vi "TestMotors.vi"() -> ()   [LabVIEW 2016]
uses:
  MotorControl/Configurations.ctl
  <vilib>/robotics/Steering/Wheel/Wheel Parameters.ctl
  <vilib>/robotics/Steering/Wheel/Rotation Direction.ctl
  <vilib>/Platform/TimedLoop/XDataNode/timing_clust.ctl
  <vilib>/Platform/TimedLoop/XDataNode/nitl_modes.ctl
  <vilib>/Platform/TimedLoop/XDataNode/wakeup.ctl
  <vilib>/myRIO/Common/Instrument Driver Framework/myRIO v1.0/UART/vis/myRIO v1.0 Close UART.vi
  <vilib>/robotics/Steering/Differential Steering Frame/NI_Robotics_Differential Steering Frame.lvclass
  C:/Program Files (x86)/National Instruments/LabVIEW 2016/vi.lib/robotics/Steering/Steering Frame/NI_Robotics_Steering Frame.lvclass
  <vilib>/robotics/Steering/Steering Frame/Apply Steering Frame Velocity to Wheels.vi
  <vilib>/myRIO/Common/Instrument Driver Framework/Utilities/vis/FPGA Ref Manager.vi
  <vilib>/myRIO/Common/Instrument Driver Framework/myRIO v1.0/myRIO v1.0 Reset FPGA.vi
  <vilib>/myRIO/Common/Instrument Driver Framework/myRIO v1.0/IRQ/vis/myRIO v1.0 IRQ Info FGV.vi
  <vilib>/myRIO/Common/Instrument Driver Framework/myRIO v1.0/IRQ/vis/myRIO v1.0 Timer IRQ Info FGV.vi
  <vilib>/myRIO/Common/Instrument Driver Framework/myRIO v1.0/IRQ/vis/myRIO v1.0 ISR Agent.vi
  <vilib>/Platform/TimedLoop/XDataNode/XDataNode.xnode
  <vilib>/Platform/TimedLoop/XDataNode/XDNodeRunTimeDep.lvlib
  <vilib>/myRIO/Instrument Drivers/Utilities/Utilities.lvlib
  <vilib>/robotics/Steering/Steering Frame/NI_Robotics_Steering Frame.lvclass
  C:/Program Files (x86)/National Instruments/LabVIEW 2016/vi.lib/robotics/Steering/Special Steering Frame/NI_Robotics_Special Steering Frame.lvclass
  <vilib>/robotics/Steering/Wheel/NI_Robotics_Wheel.lvclass
panel:
  in  "steering frame velocity":dbl[](array[numeric])=[0.0, 0.0, 0.0]
  in  "stop":bool
  out "Waveform Chart":T1(graph)
  in  "Robot Configuration":T2={"wheel parameters"={"wheel radius"=0.05, "gear ratio"=1.0, "forward rotation direction"=0}, "wheel separation"=0.19, "Encoder Pulse Per Rev"=1856.0, "Update Period (sec)"=0.02, "Initial posture frame"=[0.0, 0.0, 0.0]} {"wheel parameters"."forward rotation direction" items=["Clockwise", "Counterclockwise"]}
  out "Wheel Velocity":T5
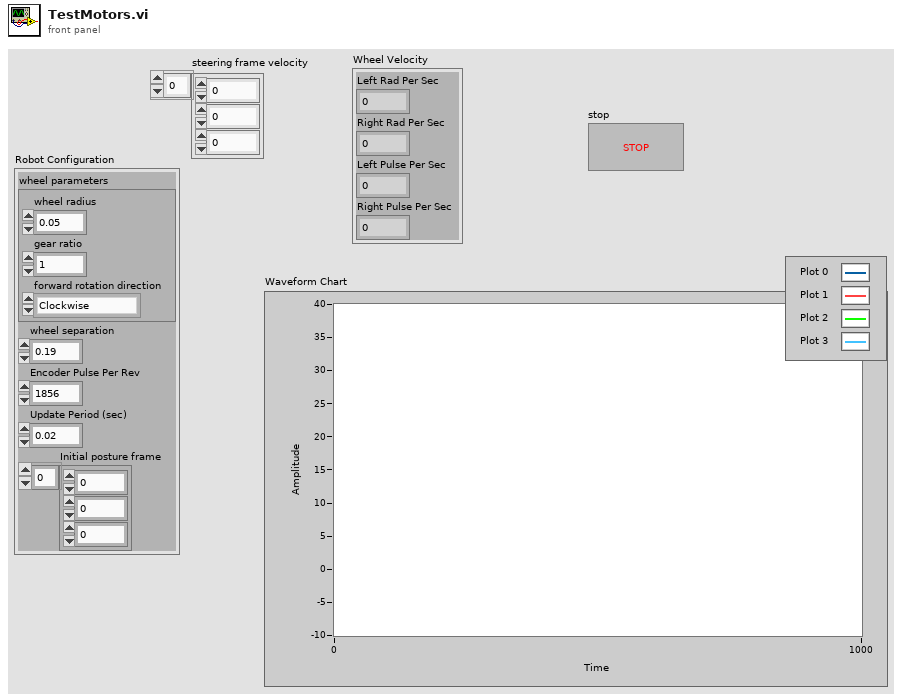
[diagram p1: front panel]
types:
  T1 = cluster{"forward angular velocity":dbl, dbl, "forward angular velocity":dbl, "Right Rad Per Sec":dbl}
  T2 = typedef "Configurations.ctl" = cluster{"wheel parameters":T3, "wheel separation":dbl, "Encoder Pulse Per Rev":dbl, "Update Period (sec)":dbl, "Initial posture frame":dbl[]}
  T3 = typedef "NI_Robotics_Wheel.lvclass/Wheel Parameters.ctl" = cluster{"wheel radius":dbl, "gear ratio":dbl, "forward rotation direction":T4}
  T4 = typedef "NI_Robotics_Wheel.lvclass/Rotation Direction.ctl" = u16
  T5 = cluster{"Left Rad Per Sec":dbl, "Right Rad Per Sec":dbl, "Left Pulse Per Sec":dbl, "Right Pulse Per Sec":dbl}
  T6 = typedef "MotorObject.ctl" = cluster{"PWM Motor Left":T7, "PWM Motor Right":T7, "DIR Motor Left":T14, "Encoder Motor Left":T17, "Encoder Motor Right":T17, "DIR Motor Right":T14, "Left DIR Forward":bool}
  T7 = typedef "PWM.lvlib/PWM Reference.ctl" = cluster{"myRIO Reference":T8, "PWM Channels Enum":T12, "PWM Configuration":T13}
  T8 = typedef "myRIO Generic Hardware Reference.ctl" = cluster{"myRIO Model":T9, "myRIO Hardware Reference":T10}
  T9 = typedef "Hardware Version Enum.ctl" = enum16{"Unknown", "myRIO-1900", "myRIO-1950", "roboRIO", "NI ELVIS RIO CM"}
  T10 = typedef "myRIO v1.0 Reference.ctl" = cluster{"Generic FPGA Reference":T11, "Allow multiple opens":bool}
  T11 = typedef "Generic FPGA Reference.ctl" = refnum<k20>
  T12 = typedef "PWM Channels Enum.ctl" = enum16{"Not Connected", "C/PWM0", "C/PWM1", "A/PWM0", "A/PWM1", "A/PWM2", "B/PWM0", "B/PWM1", "B/PWM2", "PWM/PWM0", "PWM/PWM1", "PWM/PWM2", "PWM/PWM3", "PWM/PWM4", "PWM/PWM5", "PWM/PWM6", "PWM/PWM7", "PWM/PWM8", "PWM/PWM9"}
  T13 = typedef "PWM.lvlib/PWM Configuration.ctl" = cluster{"Frequency":dbl, "Duty Cycle":dbl}
  T14 = typedef "DIO.lvlib/DIO Reference.ctl" = cluster{"myRIO Reference":T8, "DIO Channels List":T15}
  T15 = typedef "DIO Channels List.ctl" = T16[]
  T16 = typedef "DIO Channels Enum.ctl" = enum16{"Not Connected", "C/DIO0", "C/DIO1", "C/DIO2", "C/DIO3", "C/DIO4", "C/DIO5", "C/DIO6", "C/DIO7", "A/DIO0", "A/DIO1", "A/DIO2", "A/DIO3", "A/DIO4", "A/DIO5", "A/DIO6", "A/DIO7", "A/DIO8", "A/DIO9", "A/DIO10", "A/DIO11", "A/DIO12", "A/DIO13", "A/DIO14", "A/DIO15", "B/DIO0", "B/DIO1", "B/DIO2", "B/DIO3", "B/DIO4", "B/DIO5", "B/DIO6", "B/DIO7", "B/DIO8", "B/DIO9", "B/DIO10", "B/DIO11", "B/DIO12", "B/DIO13", "B/DIO14", "B/DIO15", "LED0", "LED1", "LED2", "LED3", "Button0", "DIO/DIO0", "DIO/DIO1", "DIO/DIO2", "DIO/DIO3", "DIO/DIO4", "DIO/DIO5", "DIO/DIO6", "DIO/DIO7", "DIO/DIO8", "DIO/DIO9", "SPI/CS0", "SPI/CS1", "SPI/CS2", "SPI/CS3", "LED RADIO (Green)", "LED RADIO (Red)", "LED COMM (Green)", "LED COMM (Red)", "LED MODE (Green)", "LED MODE (Red)"}
  T17 = typedef "Encoder.lvlib/Encoder Reference.ctl" = cluster{"myRIO Reference":T8, "Encoder Channels Enum":T18}
  T18 = typedef "Encoder Channels Enum.ctl" = enum16{"Not Connected", "C/ENC0", "C/ENC1", "A/ENC", "B/ENC", "DIO/ENC0", "DIO/ENC1", "DIO/ENC2", "DIO/ENC3", "DIO/ENC4"}
  T19 = typedef "XDNodeRunTimeDep.lvlib/timing_clust.ctl" = cluster{"Expected End [f-1]":u64, "Actual End [f-1]":u64, "Finished Late? [f-1]":bool, "Expected End [i-1]":u64, "Actual End [i-1]":u64, "Finished Late? [i-1]":bool, "Expected Start [i]":u64, "Actual Start [i]":u64, "Expected Start [f]":u64, "Actual Start [f]":u64, "Source Name":string, "Structure Name":string, "Period":i64, "Deadline":i64, "Offset":i64, "Start":i64, "Priority":i32, "Timeout":i32, "Mode":T20, "Wakeup Reason":T21, "Error":errorcluster, "Source Type":string, "Secondary Source Type":string, "Global End Time":u64, "Global Start Time":u64, "Frame Duration":u64, "Iteration Duration":u64, "Assigned CPU":i32, "I/O Scan Engine Mode":u32}
  T20 = typedef "XDNodeRunTimeDep.lvlib/nitl_modes.ctl" = enum32{"No Change", "Process missed periods, maintain original phase", "Discard missed periods, maintain original phase", "Process missed periods, ignore original phase", "Discard missed periods, ignore original phase"}
  T21 = typedef "XDNodeRunTimeDep.lvlib/wakeup.ctl" = enum32{"Normal", "Aborted", "Asynchronous wakeup", "Timing source error", "Timed loop error", "Timeout"}
  T22 = typedef "NI_Robotics_Wheel.lvclass/Wheel State.ctl" = cluster{"wheel name":string, "forward angular velocity":dbl, "caster angular velocity":dbl, "caster wheel angle (rad)":dbl, "steering angle (rad)":dbl}
  T23 = cluster{"forward angular velocity":dbl, "Left Rad Per Sec":dbl, "forward angular velocity":dbl, "Right Rad Per Sec":dbl}
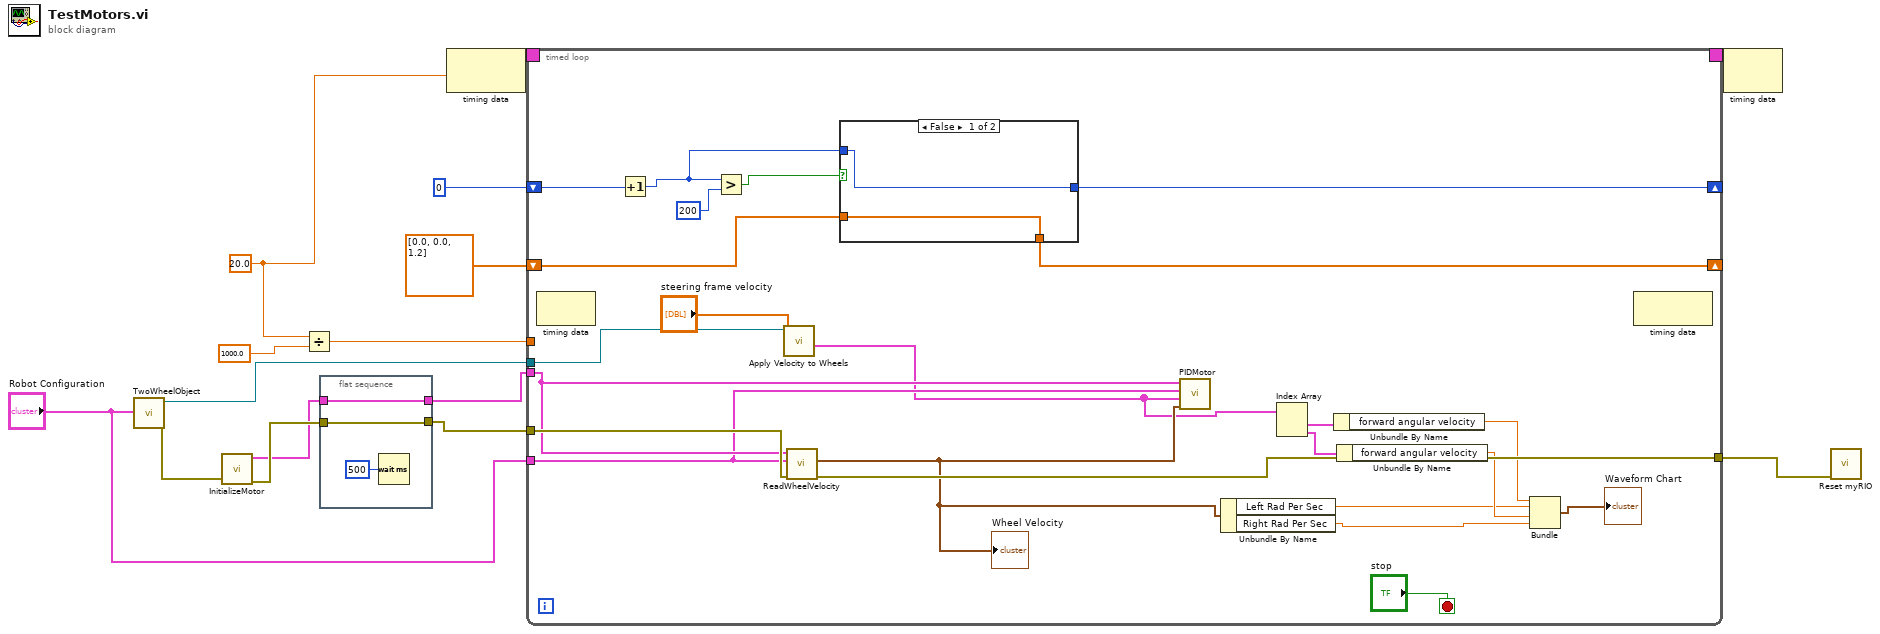
[diagram p0: block diagram]
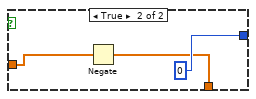
[diagram p2: hidden frame]
diagram:
  w13 = 20.0 ("Period")
  n1 = call "TwoWheelObject.vi"("Robot Configuration"="Robot Configuration") -> ("error out"=w9:errorcluster, "differential steering frame out"=w8:refnum<class "NI_Robotics_Differential Steering Frame.lvclass">)  [unwired: 9 in]
  n2 = call "InitializeMotor.vi"("error in"=w9) -> ("error out"=w7:errorcluster, "Motor Ref"=w5:T6)  [unwired: 9 in]
  n3 = Divide(x=w13, y=1000.0) -> (x/y=w11:dbl)
  n4 = flat-sequence {
    tunnel: w7 -> [w18]
    tunnel: [w18] -> w6
    tunnel: w5 -> [w16]
    tunnel: [w16] -> w4
    frame #0 {
      n5 = Wait (ms)(milliseconds to wait=u32 500) -> ()  [unwired: 1 out]
    }
  }
  n6 = node-c288(w13) -> (w15:T19)
  n7 = timed-loop {
    timing: w15 -> [_]
    timing-out: [_] -> w14
    tunnel: w6 -> [w41]
    tunnel: w4 -> [w32]
    tunnel: w11 -> [_]
    tunnel: [w40] -> w10
    tunnel: w8 -> [w39]
    shift-right: [w26] -> _
    shift-left: 0 -> [w29]
    shift-right: [w23] -> _
    shift-left: dbl[] [0.0, 0.0, 1.2] ("steering frame velocity") -> [w24]
    tunnel: "Robot Configuration" -> [w22]
    stop <- "stop" stop-if-true
    n8 = node-c288() -> ()  [unwired: 1 in, 1 out]
    n9 = Increment(x=w29) -> (x+1=w25:i32)
    n10 = Greater?(x=w25, y=200) -> (0:w27:bool)
    n11 = call-poly <vilib>:"Apply Velocity to Wheels.vi"("steering frame velocity"="steering frame velocity", "steering frame in"=w39) -> ("calculated wheel states"=w20:T22[])  [unwired: 6 in, 3 out]
    n12 = call "ReadWheelVelocity.vi"("error in"=w41, "Robot Configuration"=w22, "Motor Ref"=w32) -> ("error out"=w40:errorcluster, "Wheel Velocity"=w21:T5)  [unwired: 6 in, 1 out]
    "Wheel Velocity" <- w21
    n13 = case shown="False" w27 {
      tunnel: [w43 0] -> w26
      tunnel: w25 -> [w43 _]
      tunnel: w24 -> [w42 w45]
      tunnel: [w42 w44] -> w23
      frame False {
      }
      frame True {
        n14 = Negate(x=w45) -> (-x=w44:dbl[])
      }
    }
    n15 = call "PIDMotor.vi"("Motor Object"=w32, "Robot Configuration"=w22, "calculated wheel states"=w20, "Wheel Velocity"=w21) -> ()  [unwired: 7 in]
    n16 = Unbundle By Name(w21) -> ("Left Rad Per Sec"=w31:dbl, "Right Rad Per Sec"=w33:dbl)
    n17 = Index Array(array=w20) -> (element #1=w38:T22, element #2=w37:T22)  [unwired: 2 in]
    n18 = Unbundle By Name(w38) -> ("forward angular velocity"=w36:dbl)
    n19 = Unbundle By Name(w37) -> ("forward angular velocity"=w34:dbl)
    n20 = Bundle("forward angular velocity"=w36, "Left Rad Per Sec"=w31, "forward angular velocity"=w34, "Right Rad Per Sec"=w33) -> (→"Waveform Chart":T23)  [unwired: 1 in]
    n21 = node-c288() -> ()  [unwired: 1 in, 1 out]
  }
  n22 = node-c288(w14) -> ()  [unwired: 1 out]
  n23 = call <vilib>:"Reset myRIO.vi"("error in (no error)"=w10) -> ()  [unwired: 10 in, 1 out]
